vi "LNLS Control Receive Command Body.vi"(8 "error in (no error)":errorcluster, 10 "timeout ms (10000)":i32=10000, 11 "connection ID":refnum<k5>) -> (0 "error out":errorcluster, 1 "command length":u8, 2 "command body":string, 3 "connection ID out":refnum<k5>)   [LabVIEW 2011, in "LNLS Control VIs.lvlib"]
uses:
  LNLS Control VIs.lvlib
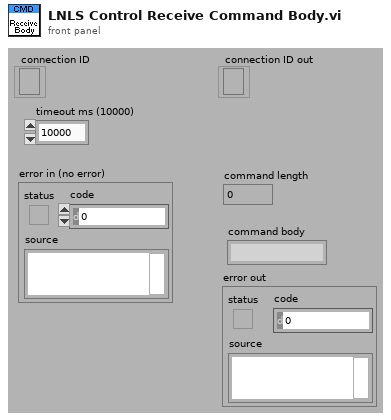
[diagram p1: front panel]
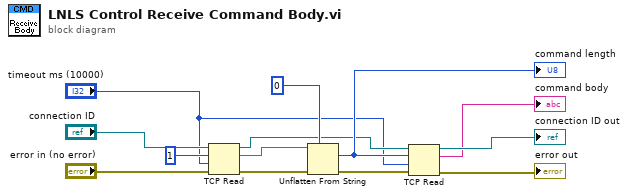
[diagram p0: block diagram]
diagram:
  n1 = TCP Read(connection ID="connection ID", bytes to read=1, error in (no error)="error in (no error)", 9:"timeout ms (10000)") -> (connection ID out=w5:refnum<k5>, data out=w2:string, error out=w3:errorcluster)  [unwired: 1 in]
  n2 = Unflatten From String(type=u8 0 ("length"), binary string=w2, error in (no error)=w3) -> (value=w11:u8, error out=w4:errorcluster)  [unwired: 2 in, 1 out]
  "command length" <- w11
  n3 = TCP Read(connection ID=w5, bytes to read=w11, error in (no error)=w4, 9:"timeout ms (10000)") -> (connection ID out=→"connection ID out":refnum<k5>, data out=→"command body":string, error out=→"error out":errorcluster)  [unwired: 1 in]
